vi "Index Waveform Array Elements.vi"(9 "Indices of Elements":i32[](array[numeric]), 11 "Array in":waveform(dbl)[](array[waveform])) -> (3 "Array out":waveform(dbl)[](array[waveform]))   [LabVIEW 2019, in "DSP.lvclass"]
uses:
  DSP.lvclass
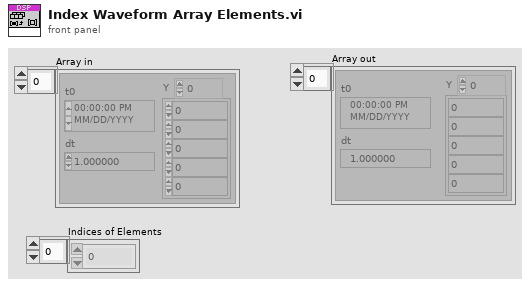
[diagram p1: front panel]
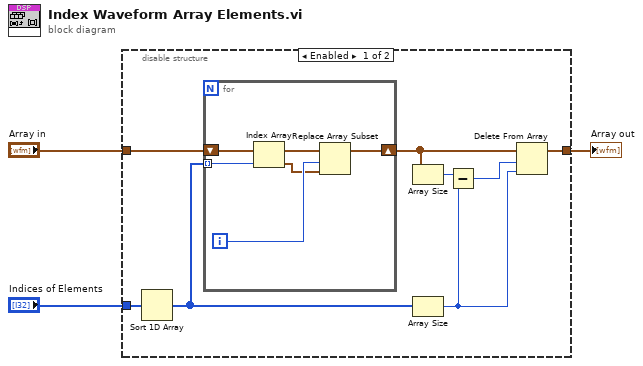
[diagram p0: block diagram]
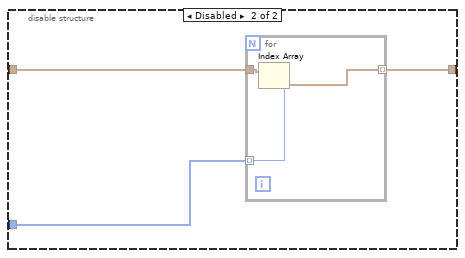
[diagram p2: hidden frame]
diagram:
  n1 = disable-structure shown="Enabled" {
    disable-tunnel: "Array in" -> [w11 w19]
    disable-tunnel: "Indices of Elements" -> [w10 w18]
    disable-tunnel: [w9 w17] -> w1
    frame Enabled {
      n2 = Sort 1D Array(array=w10) -> (sorted array=w7:i32[])
      n3 = for {
        tunnel: w7 -> [w16] mode=indexing
        shift-right: [w15] -> w8
        shift-left: w11 -> [w14]
        i -> [w13]
        n4 = Index Array(array=w14, index=w16) -> (element=w12:waveform(dbl))
        n5 = Replace Array Subset(array=w14, new element=w12, index=w13) -> (w15:waveform(dbl)[])
      }
      n6 = Array Size(array=w8) -> (size(s)=w6:i32)
      n7 = Array Size(array=w7) -> (size(s)=w4:i32)
      n8 = Subtract(x=w6, y=w4) -> (x-y=w5:i32)
      n9 = Delete From Array(array=w8, length=w5, index=w4) -> (array with subset deleted=w9:waveform(dbl)[])  [unwired: 1 out]
    }
    frame Disabled {
      n10 = for {
        tunnel: w19 -> [w22]
        tunnel: w18 -> [w21] mode=indexing
        tunnel: [w20] -> w17 mode=indexing
        n11 = Index Array(array=w22, index=w21) -> (element=w20:waveform(dbl))
      }
    }
  }
  "Array out" <- w1
